vi "testLoopback.vi"(8 "error in (no error)":errorcluster, 11 "TestCase in":refnum<class "SLSC 12201 System Tests.lvclass">) -> (0 "error out":errorcluster, 3 "TestCase out":refnum<class "SLSC 12201 System Tests.lvclass">)   [LabVIEW 2015, in "SLSC 12201 System Tests.lvclass"]
uses:
  SLSC 12201 System Tests.lvclass
  niveristand-custom-device-testing-tools/Loopback/Loopback.lvclass
  <vilib>/addons/_JKI Toolkits/VI Tester/TestCase.llb/TestCase.lvclass
  niveristand-custom-device-testing-tools/VeriStandTestCase/VeriStandTestCase.lvclass
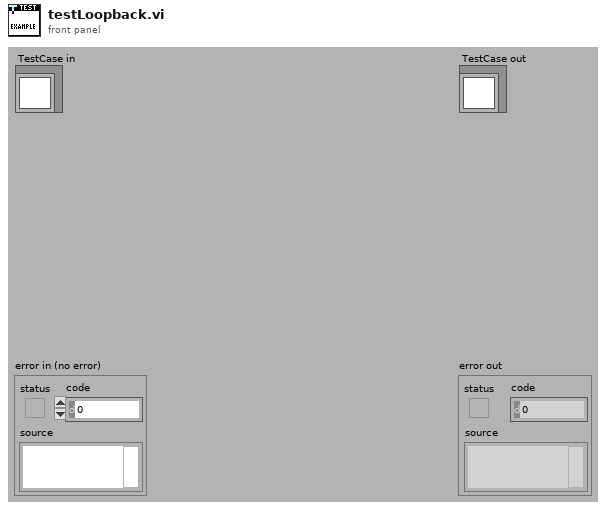
[diagram p1: front panel]
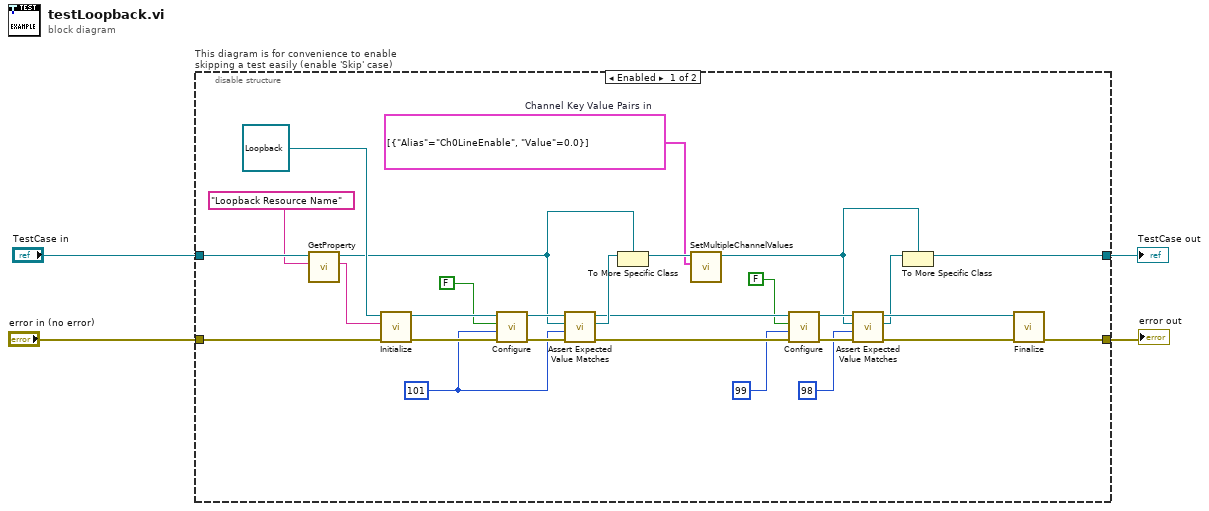
[diagram p0: block diagram]
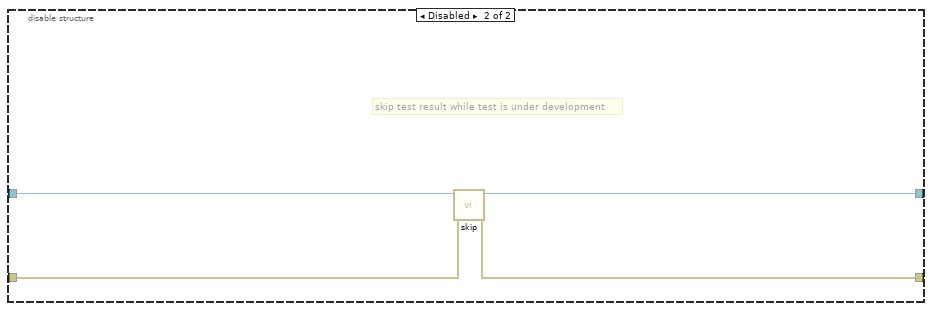
[diagram p2: hidden frame]
diagram:
  n1 = disable-structure "This diagram is for convenience to enable skipping a test easily (enable 'Skip' case)" shown="Enabled" {
    disable-tunnel: "TestCase in" -> [w30 w34]
    disable-tunnel: [w6 w32] -> w1
    disable-tunnel: [w26 w33] -> w3
    disable-tunnel: "error in (no error)" -> [w29 w31]
    frame Enabled {
      w13 = cluster{"Alias":string, "Value":dbl}[] [{"Alias"="Ch0LineEnable", "Value"=0.0}]  # Channel Key Value Pairs in
      w17 = u8 101 ("Value in")
      n2 = call "GetProperty.vi"("key"="Loopback Resource Name", "VeriStandTestCase in"=w30) -> ("value"=w24:string, "VeriStandTestCase out"=w15:refnum<class "SLSC 12201 System Tests.lvclass">)  [unwired: 7 in, 1 out]
      n3 = call-dynamic "Initialize.vi"("error in (no error)"=w29, "Resource Name in"=w24, "Loopback in"=refnum<class "Loopback.lvclass"> refnum ("Loopback.lvclass")) -> ("error out"=w27:errorcluster, "Loopback out"=w22:refnum<class "Loopback.lvclass">)  [unwired: 7 in]
      n4 = call-dynamic "Configure.vi"("error in (no error)"=w27, "Value in"=w17, "Use Counter?"=FALSE, "Loopback in"=w22) -> ("error out"=w23:errorcluster, "Loopback out"=w19:refnum<class "Loopback.lvclass">)  [unwired: 6 in]
      n5 = call-dynamic "Assert Expected Value Matches.vi"("error in (no error)"=w23, "Expected Value"=w17, "TestCase in"=w15, "Loopback in"=w19) -> ("error out"=w20:errorcluster, "TestCase out"=w18:refnum<class "TestCase.lvclass">, "Loopback out"=w14:refnum<class "Loopback.lvclass">)  [unwired: 5 in]
      n6 = To More Specific Class(target class=w15, reference=w18) -> (specific class reference=w16:refnum<class "SLSC 12201 System Tests.lvclass">)  [unwired: 1 in, 1 out]
      n7 = call-dynamic "SetMultipleChannelValues.vi"("Channel Key Value Pairs in"=w13, "VeriStandTestCase in"=w16) -> ("VeriStandTestCase out"=w5:refnum<class "SLSC 12201 System Tests.lvclass">)  [unwired: 8 in, 1 out]
      n8 = call-dynamic "Configure.vi"("Value in"=u8 99, "Use Counter?"=FALSE, "Loopback in"=w14) -> ("Loopback out"=w12:refnum<class "Loopback.lvclass">)  [unwired: 7 in, 1 out]
      n9 = call-dynamic "Assert Expected Value Matches.vi"("Expected Value"=u8 98, "TestCase in"=w5, "Loopback in"=w12) -> ("TestCase out"=w7:refnum<class "TestCase.lvclass">, "Loopback out"=w9:refnum<class "Loopback.lvclass">)  [unwired: 6 in, 1 out]
      n10 = To More Specific Class(target class=w5, reference=w7) -> (specific class reference=w6:refnum<class "SLSC 12201 System Tests.lvclass">)  [unwired: 1 in, 1 out]
      n11 = call-dynamic "Finalize.vi"("error in (no error)"=w20, "Loopback in"=w9) -> ("error out"=w26:errorcluster)  [unwired: 8 in, 1 out]
    }
    frame Disabled {
      # "skip test result while test is under development"
      n12 = call <vilib>:"skip.vi"("error in (no error)"=w31, "TestCase in"=w34) -> ("error out"=w33:errorcluster, "TestCase out"=w32:refnum<class "SLSC 12201 System Tests.lvclass">)  [unwired: 8 in]
    }
  }
  "error out" <- w3
  "TestCase out" <- w1
